vi "Panel.vi"() -> ()   [LabVIEW 2011]
uses:
  Laba3/Global.vi
  <vilib>/Utility/file.llb/Write To Spreadsheet File (string).vi
panel:
  out "Ёмкость 2":dbl(slide) scale=0.0..100.0
  out "Термометр 2":dbl(slide) scale=0.0..50.0
  in  "Tab Control":enum32{"Параметры", "График", "Таблица"}(tab)
  out "Температура":dbl
  out "Уровень":dbl
  out "Ёмкость":dbl(slide) scale=0.0..100.0
  out "Термометр":dbl(slide) scale=0.0..50.0
  out "Waveform Chart":cluster{"Temp":dbl, "Level":dbl}(graph)
  out "Table Control":string[][](table)
  in  "stop":bool
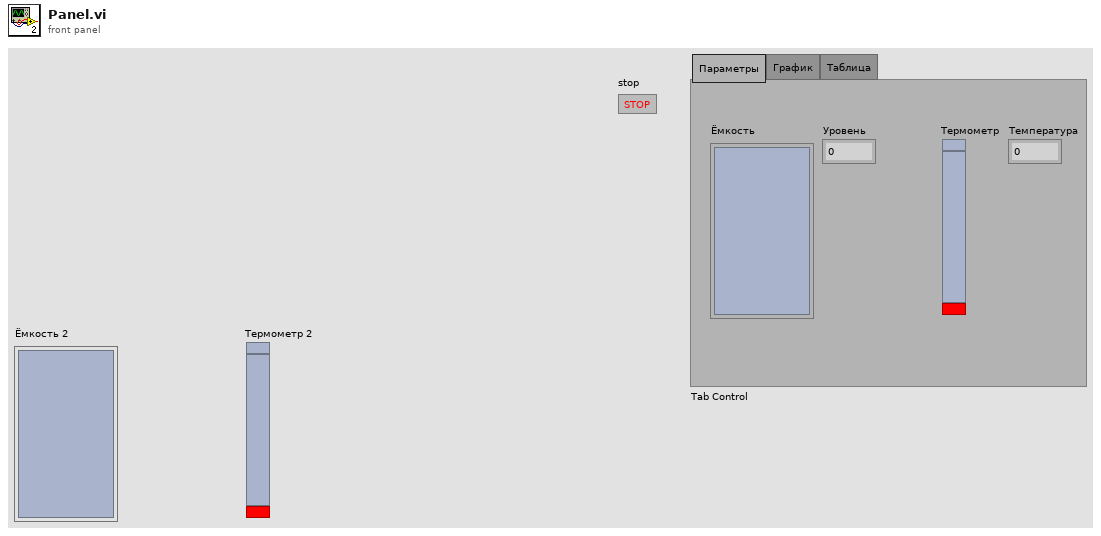
[diagram p1: front panel]
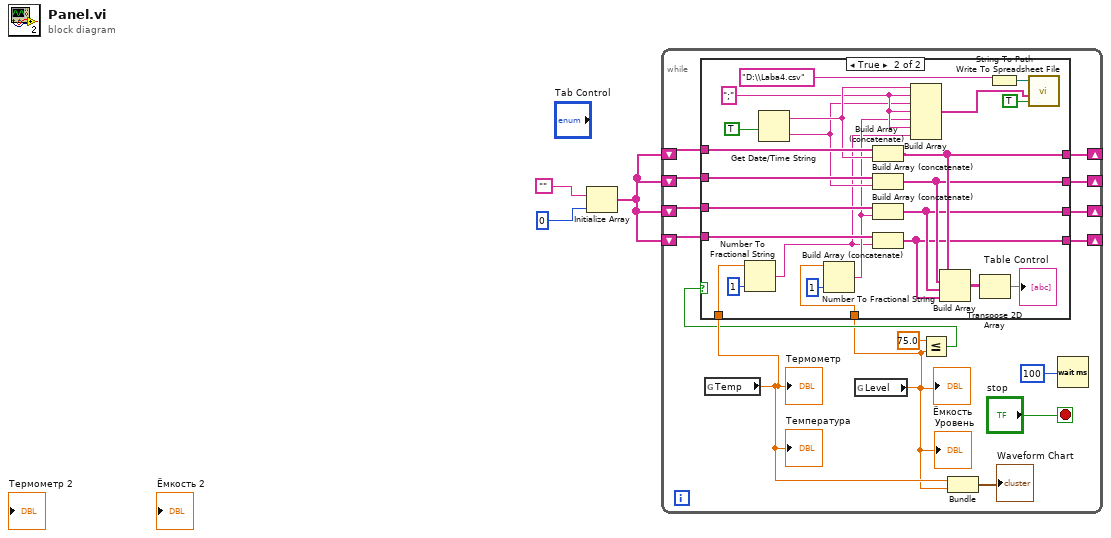
[diagram p0: block diagram]
diagram:
  n1 = Initialize Array("", 0) -> (w3:string[])
  n2 = while {
    shift-right: [w15] -> _
    shift-left: w3 -> [w11]
    shift-right: [w14] -> _
    shift-left: w3 -> [w10]
    shift-right: [w13] -> _
    shift-left: w3 -> [w9]
    shift-right: [w12] -> _
    shift-left: w3 -> [w8]
    stop <- "stop" stop-if-true
    n3 = global read "Global.vi" "Temp"() -> (w7:dbl)
    "Термометр" <- w7
    "Температура" <- w7
    n4 = global read "Global.vi" "Level"() -> (w5:dbl)
    "Ёмкость" <- w5
    "Уровень" <- w5
    n5 = Less Or Equal?(x=75.0, y=w5) -> (x <= y?=w6:bool)
    n6 = case shown="True" w6 {
      tunnel: [w22 w40] -> w15
      tunnel: [w21 w39] -> w14
      tunnel: [w20 w38] -> w13
      tunnel: [w19 w37] -> w12
      tunnel: w11 -> [w22 w46]
      tunnel: w10 -> [w21 w45]
      tunnel: w9 -> [w20 w44]
      tunnel: w8 -> [w19 w43]
      tunnel: w7 -> [_ w36]
      tunnel: w5 -> [_ w35]
      frame False {
      }
      frame True {
        w27 = ";"
        n7 = Number To Fractional String(number=w36, precision (6)=1) -> (F-format string=w24:string)  [unwired: 2 in]
        n8 = Get Date/Time String(want seconds? (F)=TRUE) -> (date string=w28:string, time string=w26:string)  [unwired: 2 in]
        n9 = Number To Fractional String(number=w35, precision (6)=1) -> (F-format string=w25:string)  [unwired: 2 in]
        n10 = Build Array (concatenate)(w46, w28) -> (w40:string[])
        n11 = Build Array (concatenate)(w45, w26) -> (w39:string[])
        n12 = Build Array (concatenate)(w44, w25) -> (w38:string[])
        n13 = Build Array (concatenate)(w43, w24) -> (w37:string[])
        n14 = Build Array(w28, w27, w26, w27, w25, w27, w24) -> (w29:string[])
        n15 = Build Array(w40, w39, w38, w37) -> (w41:string[][])
        n16 = Transpose 2D Array(2D array=w41) -> (transposed array=→"Table Control":string[][])
        n17 = String To Path(string="D:\\Laba4.csv") -> (path=w30:path)
        n18 = call-poly <vilib>:"Write To Spreadsheet File.vi"("append to file? (new file:F)"=TRUE, "1D data"=w29, "file path (dialog if empty)"=w30) -> ()  [unwired: 5 in, 1 out]
      }
    }
    n19 = Bundle("Temp"=w7, "Level"=w5) -> (→"Waveform Chart":cluster{"Temp":dbl, "Level":dbl})  [unwired: 1 in]
    n20 = Wait (ms)(milliseconds to wait=100) -> ()  [unwired: 1 out]
  }
